vi "File.Date String, File Safe.vi"() -> (1 "Date":string)   [LabVIEW 2018]
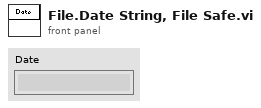
[diagram p1: front panel]
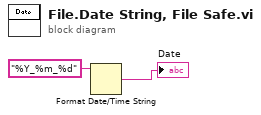
[diagram p0: block diagram]
diagram:
  n1 = Format Date/Time String(time format string (%c)="%Y_%m_%d") -> (date/time string=→"Date":string)  [unwired: 2 in]
